vi "K2420 current from bias pulse.vi"() -> ()   [LabVIEW 2014]
uses:
  <vilib>/Utility/file.llb/Write To Spreadsheet File (string).vi
  Environmental Chamber LabVIEW and Instruments/Drivers and Software/LabVIEW 8.2 Drivers/keithley_24xx/Keithley 24XX/Public/Data/Read (Single Point).vi
  Environmental Chamber LabVIEW and Instruments/Drivers and Software/keithley_24xx/Keithley 24XX/Keithley 24XX.lvlib
panel:
  out "Resistance":sgl
  out "Current":sgl
  out "Voltage":sgl
  out "XY Graph":cluster{"X":dbl[], "Y":dbl[]}[](graph)
  in  "Voltage Output Level":dbl=0.01
  in  "save?":bool
  in  "note":string
  in  "Stop Button":bool
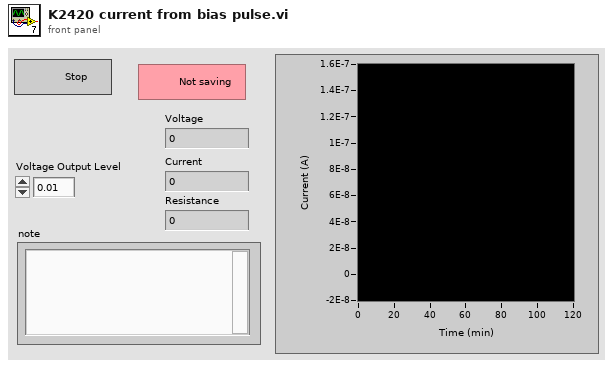
[diagram p1: front panel]
types:
  T1 = enum16{"open", "open or create", "create or replace", "create", "open (read only)"}
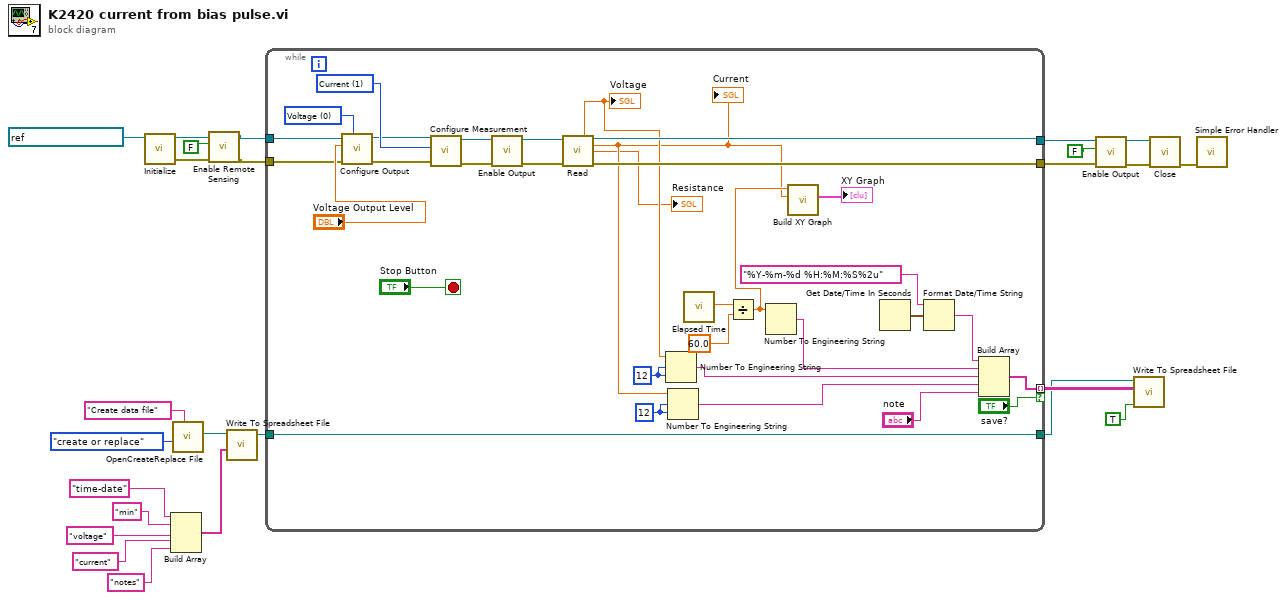
[diagram p0: block diagram]
diagram:
  n1 = call "Initialize.vi"("VISA resource name"=refnum<visa-resource-name> "GPIB1::24::INSTR") -> ("error out"=w19:errorcluster, "VISA resource name out"=w20:refnum<visa-resource-name>)  [unwired: 9 in]
  n2 = Build Array("time-date" ("note 2"), "min" ("note 2"), "voltage" ("note 2"), "current" ("note 2"), "notes" ("note 2")) -> (w7:string[])
  n3 = call "OpenCreateReplace File.vi"("prompt"="Create data file", "function (open:0)"=T1."create or replace") -> ("new file path"=w8:path)  [unwired: 6 in, 3 out]
  n4 = call "Enable Remote Sensing.vi"("error in (no error)"=w19, "Enable Remote Sensing (T: Enable)"=FALSE ("4-wire?"), "VISA resource name"=w20) -> ("error out"=w3:errorcluster, "VISA resource name out"=w4:refnum<visa-resource-name>)  [unwired: 7 in]
  n5 = call-poly <vilib>:"Write To Spreadsheet File.vi"("1D data"=w7, "file path (dialog if empty)"=w8) -> ("new file path (Not A Path if cancelled)"=w6:path)  [unwired: 6 in]
  n6 = while {
    tunnel: [w56] -> w23 mode=indexing if="save?"
    tunnel: w4 -> [w37]
    tunnel: w3 -> [w35]
    tunnel: [w48] -> w5
    tunnel: w6 -> [w48]
    tunnel: [w52] -> w13
    tunnel: [w51] -> w12
    stop <- "Stop Button" stop-if-true
    w31 = i16 12 ("width (-)")
    w43 = u16 0 items=["Voltage", "Current"] ("Source")
    w38 = u16 1 items=["Volts", "Current", "Resistance"] ("Measure")
    w53 = i16 12 ("width (-)")
    n7 = call "Configure Output.vi"("Source Mode  (0: Voltage)"=w43, "error in (no error)"=w35, "Output Level (0)"="Voltage Output Level", "VISA resource name"=w37) -> ("error out"=w34:errorcluster, "VISA resource name out"=w36:refnum<visa-resource-name>)  [unwired: 6 in]
    n8 = call "Configure Measurement.vi"("error in (no error)"=w34, "Function (0: Volts)"=w38, "VISA resource name"=w36) -> ("error out"=w33:errorcluster, "VISA resource name out"=w32:refnum<visa-resource-name>)  [unwired: 7 in]
    n9 = call "Enable Output.vi"("error in (no error)"=w33, "VISA resource name"=w32) -> ("error out"=w41:errorcluster, "VISA resource name out"=w42:refnum<visa-resource-name>)  [unwired: 8 in]
    n10 = call-poly "Read.vi"("VISA resource name"=w42, "error in (no error)"=w41) -> ("Voltage"=w28:sgl, "VISA resource name out"=w52:refnum<visa-resource-name>, "Current"=w27:sgl, "Resistance"=→"Resistance":sgl, "error out"=w51:errorcluster)  [unwired: 7 in, 2 out]
    "Voltage" <- w28
    "Current" <- w27
    n11 = Number To Engineering String(2:w53, 3:w53, 4:w28) -> (0:w46:string)  [unwired: 1 in]
    n12 = Number To Engineering String(2:w31, 3:w31, 4:w27) -> (0:w29:string)  [unwired: 1 in]
    n13 = call "Elapsed Time"() -> ("Elapsed Time (s)"=w50:dbl)  [unwired: 12 in, 7 out]
    n14 = Divide(x=w50, y=60.0) -> (x/y=w39:dbl)
    n15 = Number To Engineering String ("elapsed time (min)")(4:w39) -> (0:w54:string)  [unwired: 3 in]
    n16 = call "Build XY Graph"("Y Input"=w27, "X Input"=w39) -> ("XY Graph"=→"XY Graph":cluster{"X":dbl[], "Y":dbl[]}[])  [unwired: 8 in, 1 out]
    n17 = Get Date/Time In Seconds() -> (seconds since 1Jan1904=w58:timestamp)
    n18 = Format Date/Time String(time format string (%c)="%Y-%m-%d %H:%M:%S%2u", seconds (now)=w58) -> (date/time string=w55:string)  [unwired: 1 in]
    n19 = Build Array(w55, w54, w46, w29, "note") -> (w56:string[])
  }
  n20 = call "Enable Output.vi"("error in (no error)"=w12, "Enable Output (T: Enable)"=FALSE, "VISA resource name"=w13) -> ("error out"=w15:errorcluster, "VISA resource name out"=w17:refnum<visa-resource-name>)  [unwired: 7 in]
  n21 = call-poly <vilib>:"Write To Spreadsheet File.vi"("append to file? (new file:F)"=TRUE, "2D data"=w23, "file path (dialog if empty)"=w5) -> ()  [unwired: 5 in, 1 out]
  n22 = call "Close.vi"("error in (no error)"=w15, "VISA resource name"=w17) -> ("error out"=w14:errorcluster)  [unwired: 9 in]
  n23 = call <vilib>:"Simple Error Handler.vi"("error in (no error)"=w14) -> ()  [unwired: 4 in, 5 out]
